vi "SetOperationMode_old.vi"(0 "VISA resource name in":refnum<visa-resource-name>, 5 "ON/OFF":bool, 9 "Operation Mode Status":T1, 11 "error in":errorcluster, 12 "Laser":bool) -> (4 "VISA resource name out":refnum<visa-resource-name>, 10 "Message":string, 15 "error out":errorcluster)   [LabVIEW 2014]
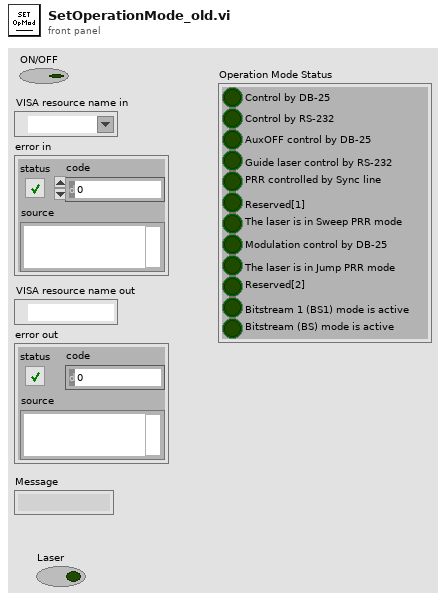
[diagram p1: front panel]
types:
  T1 = cluster{"Control by DB-25":bool, "Control by RS-232":bool, "AuxOFF control by DB-25":bool, "Guide laser control by RS-232":bool, "PRR controlled by Sync line ":bool, "Reserved[1]":bool, "The laser is in Sweep PRR mode":bool, "Modulation control by DB-25":bool, "The laser is in Jump PRR mode":bool, "Reserved[2]":bool, "Bitstream 1 (BS1) mode is active":bool, "Bitstream (BS) mode is active":bool}
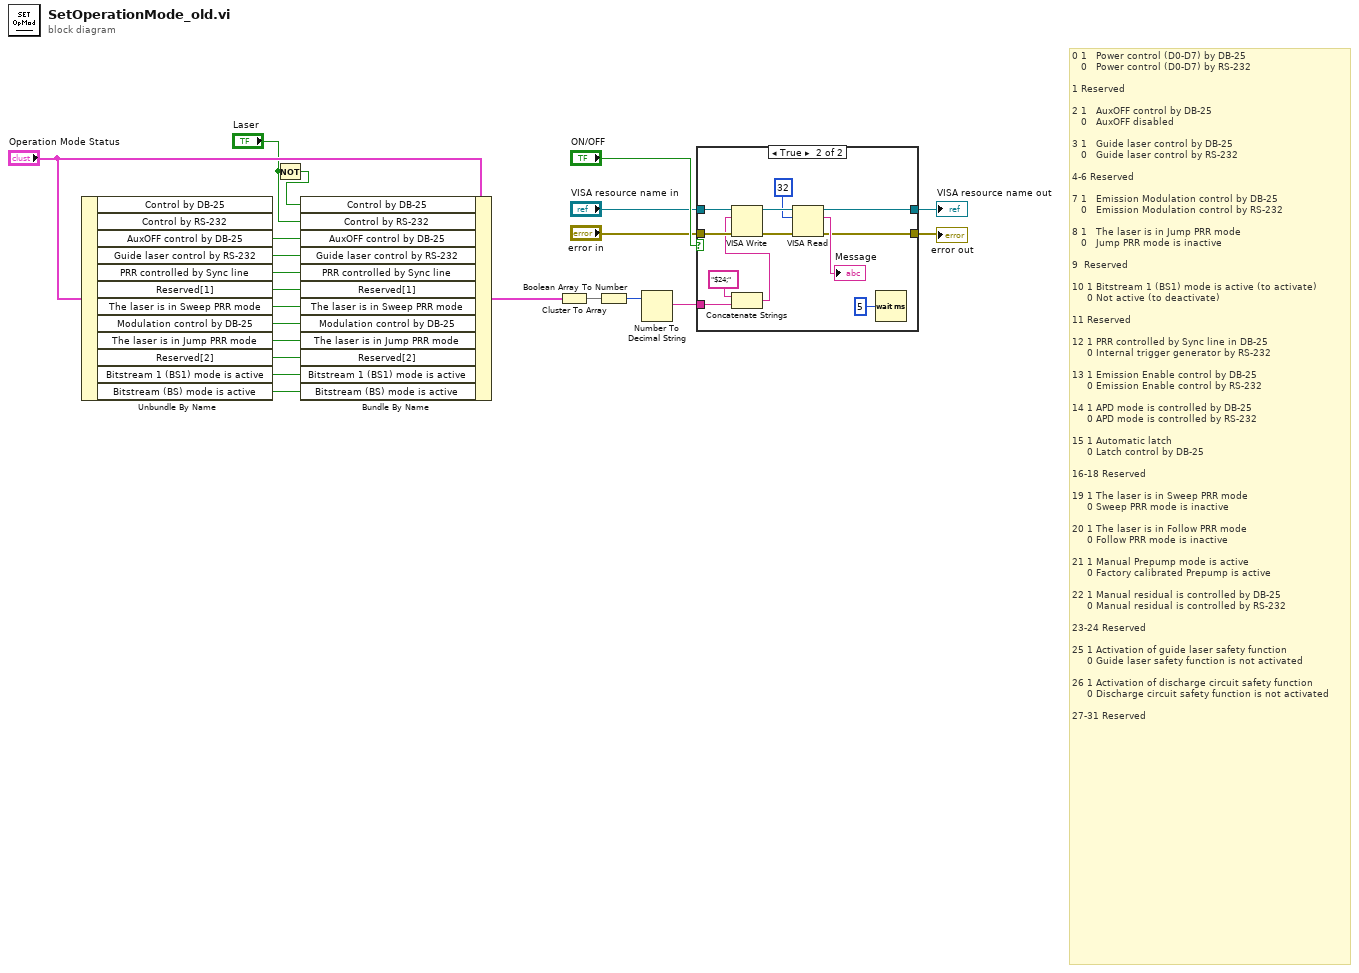
[diagram p0: block diagram]
diagram:
  # "0 1   Power control (D0-D7) by DB-25\n   0   Power control (D0-D7) by RS-232\n\n1 Reserved\n\n2 1   AuxOFF control by DB-25\n   0   AuxOFF disabled\n\n3 1   Guide laser control by DB-25\n   0   Guide laser control by RS-232\n\n4-6 Reserved\n\n7 1   Emission Modulation control by DB-25\n   0   Emission Modulation control by RS-232\n\n8 1   The laser is in Jump PRR mode\n   0   Jump PRR mode is inactive\n\n9  Reserved\n\n10 1 Bitstream 1 (BS1) mode is active (to activate)\n     0 Not active (to deactivate)\n\n11 Reserved\n\n12 1 PRR controlled by Sync line in DB-25\n     0 Internal trigger generator by RS-232\n\n13 1 Emission Enable control by DB-25\n     0 Emission Enable control by RS-232\n\n14 1 APD mode is controlled by DB-25\n     0 APD mode is controlled by RS-232\n\n15 1 Automatic latch\n     0 Latch control by DB-25\n\n16-18 Reserved\n\n19 1 The laser is in Sweep PRR mode\n     0 Sweep PRR mode is inactive\n\n20 1 The laser is in Follow PRR mode\n     0 Follow PRR mode is inactive\n\n21 1 Manual Prepump mode is active\n     0 Factory calibrated Prepump is active\n\n22 1 Manual residual is controlled by DB-25\n     0 Manual residual is controlled by RS-232\n\n23-24 Reserved\n\n25 1 Activation of guide laser safety function\n     0 Guide laser safety function is not activated\n\n26 1 Activation of discharge circuit safety function\n     0 Discharge circuit safety function is not activated\n\n27-31 Reserved"
  n1 = Unbundle By Name("Operation Mode Status") -> ("AuxOFF control by DB-25"=w13:bool, "Guide laser control by RS-232"=w3:bool, "PRR controlled by Sync line"=w12:bool, "Reserved[1]"=w11:bool, "The laser is in Sweep PRR mode"=w10:bool, "Modulation control by DB-25"=w1:bool, "The laser is in Jump PRR mode"=w9:bool, "Reserved[2]"=w8:bool, "Bitstream 1 (BS1) mode is active"=w7:bool, "Bitstream (BS) mode is active"=w6:bool)  [unwired: 2 out]
  n2 = Not(x="Laser") -> (.not. x?=w2:bool)
  n3 = Bundle By Name(cluster="Operation Mode Status", "Control by DB-25"=w2, "Control by RS-232"="Laser", "AuxOFF control by DB-25"=w13, "Guide laser control by RS-232"=w3, "PRR controlled by Sync line"=w12, "Reserved[1]"=w11, "The laser is in Sweep PRR mode"=w10, "Modulation control by DB-25"=w1, "The laser is in Jump PRR mode"=w9, "Reserved[2]"=w8, "Bitstream 1 (BS1) mode is active"=w7, "Bitstream (BS) mode is active"=w6) -> (w5:T1)
  n4 = Cluster To Array(cluster=w5) -> (array=w14:bool[])
  n5 = Boolean Array To Number(Boolean array=w14) -> (number=w17:u32)
  n6 = Number To Decimal String(number=w17) -> (decimal integer string=w16:string)  [unwired: 1 in]
  n7 = case shown="True" "ON/OFF" {
    tunnel: "VISA resource name in" -> [w24 w34]
    tunnel: "error in" -> [w23 w33]
    tunnel: [w24 w26] -> w19
    tunnel: [w23 w25] -> w18
    tunnel: w16 -> [_ w28]
    frame False {
    }
    frame True {
      n8 = Concatenate Strings("$24;" ("write buffer"), w28) -> (w27:string)
      n9 = VISA Write(VISA resource name=w34, write buffer=w27, error in (no error)=w33) -> (VISA resource name out=w35:refnum<visa-resource-name>, error out=w36:errorcluster)  [unwired: 1 out]
      n10 = VISA Read(VISA resource name=w35, byte count=u32 32, error in (no error)=w36) -> (VISA resource name out=w26:refnum<visa-resource-name>, read buffer=→"Message":string, error out=w25:errorcluster)  [unwired: 1 out]
      n11 = Wait (ms)(milliseconds to wait=u32 5) -> ()  [unwired: 1 out]
    }
  }
  "VISA resource name out" <- w19
  "error out" <- w18
